vi "ConfigurationPage.vi"(9 "Parameter defaults":string, 10 "Parameters":T1, 11 "Stop":T2) -> ()   [LabVIEW 2020, in "DefaultExtensions.lvlib" / "CGrapherDGML.lvclass"]
uses:
  CGrapherDGML.lvclass
  Private/Parameters.ctl
  obj/Addons/ExtensionInterfaces.lvlibp/IConfigurationPage/Event_Stop.ctl
  obj/Addons/ExtensionInterfaces.lvlibp/IConfigurationPage/IConfigurationPage.lvclass
  obj/Addons/ExtensionInterfaces.lvlibp/IConfigurationPage/Event_StopRef.ctl
  obj/Addons/ExtensionInterfaces.lvlibp/IConfigurationPage/Event_Parameters.ctl
  obj/Addons/ExtensionInterfaces.lvlibp/IConfigurationPage/Event_ParametersRef.ctl
panel:
  in  "Add virtual folders?":bool
  in  "Group by folder":bool
  in  "Expand containers":bool
  in  "Show full paths":bool
  in  "Source folder?":bool
  in  "Target folder?":bool
  in  "Results path":path
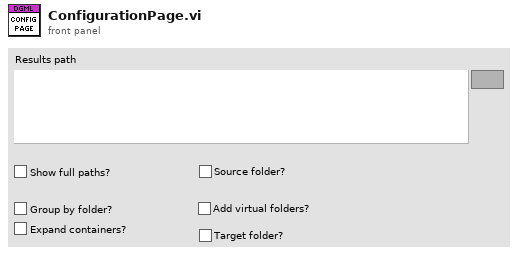
[diagram p1: front panel]
types:
  T1 = typedef "ExtensionInterfaces.lvlibp/IConfigurationPage.lvclass/Event_ParametersRef.ctl" = refnum<user-event>
  T2 = typedef "ExtensionInterfaces.lvlibp/IConfigurationPage.lvclass/Event_StopRef.ctl" = refnum<user-event>
  T3 = typedef "DefaultExtensions.lvlib/CGrapherDGML.lvclass/Parameters.ctl" = cluster{"Path":string, "Expand containers":bool, "Group by folder":bool, "Show full paths":bool, "Source folder?":bool, "Target folder?":bool, "Add virtual folders?":bool}
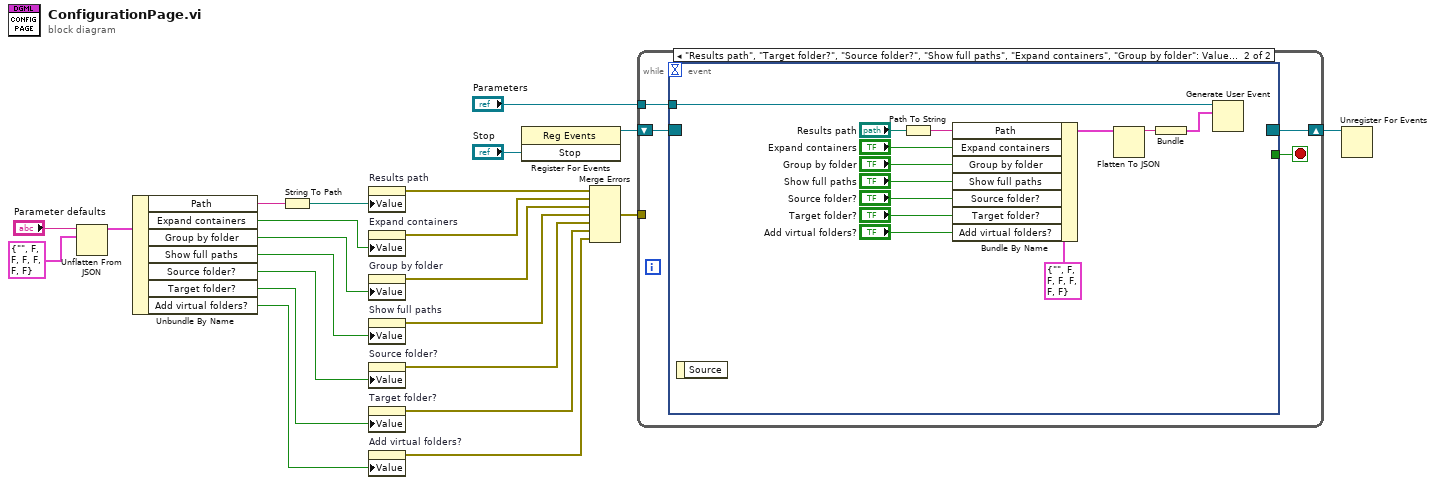
[diagram p0: block diagram]
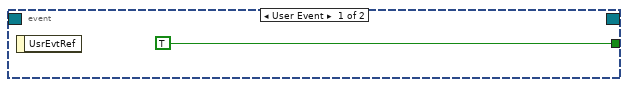
[diagram p2: hidden frame]
diagram:
  n1 = Unflatten From JSON(JSON string="Parameter defaults", type and defaults=T3 {"Path"="", "Expand containers"=FALSE, "Group by folder"=FALSE, "Show full paths"=FALSE, "Source folder?"=FALSE, "Target folder?"=FALSE, "Add virtual folders?"=FALSE} ("Parameters")) -> (value=w17:T3)  [unwired: 5 in, 1 out]
  n2 = Unbundle By Name(w17) -> ("Path"=w16:string, "Expand containers"=w14:bool, "Group by folder"=w13:bool, "Show full paths"=w12:bool, "Source folder?"=w11:bool, "Target folder?"=w10:bool, "Add virtual folders?"=w1:bool)
  n3 = String To Path(string=w16) -> (path=w15:path)
  n4 = property on="Results path" class="Path"("Value"=w15) -> (error out=w9:errorcluster)  [unwired: 2 in, 1 out]
  n5 = property on="Expand containers" class="Bool (strict)"("Value"=w14) -> (error out=w8:errorcluster)  [unwired: 2 in, 1 out]
  n6 = property on="Group by folder" class="Bool (strict)"("Value"=w13) -> (error out=w7:errorcluster)  [unwired: 2 in, 1 out]
  n7 = property on="Show full paths" class="Bool (strict)"("Value"=w12) -> (error out=w6:errorcluster)  [unwired: 2 in, 1 out]
  n8 = property on="Source folder?" class="Bool (strict)"("Value"=w11) -> (error out=w5:errorcluster)  [unwired: 2 in, 1 out]
  n9 = property on="Target folder?" class="Bool (strict)"("Value"=w10) -> (error out=w4:errorcluster)  [unwired: 2 in, 1 out]
  n10 = property on="Add virtual folders?" class="Bool (strict)"("Value"=w1) -> (error out=w2:errorcluster)  [unwired: 2 in, 1 out]
  n11 = register-events("Stop") -> (reference out=w23:refnum<event-registration>)  [unwired: 2 in, 1 out]
  n12 = Merge Errors(w9, w8, w7, w6, w5, w4, w2) -> (w3:errorcluster)
  n13 = while {
    shift-right: [w26] -> w22
    shift-left: w23 -> [w27]
    tunnel: "Parameters" -> [w24]
    tunnel: w3 -> [_]
    stop <- w25 stop-if-true
    n14 = event shown="[1] \"Results path\", \"Target folder?\", \"Source folder?\", \"Show full paths\", \"Expand containers\", \"Group by folder\": Value Change" {
      selector: w27 -> [_ _]
      dyn-events: [_ _] -> w26
      timeout: _ -> [_ _]
      tunnel: [TRUE _] -> w25
      tunnel: w24 -> [_ w37]
      event User Event {
        n15 = event-data() -> ()  [unwired: 1 in, 1 out]
      }
      event "Results path", "Target folder?", "Source folder?", "Show full paths", "Expand containers", "Group by folder": Value Change {
        n16 = event-data() -> ()  [unwired: 1 in, 1 out]
        n17 = Path To String(path="Results path") -> (string=w40:string)
        n18 = Bundle By Name(cluster=T3 {"Path"="", "Expand containers"=FALSE, "Group by folder"=FALSE, "Show full paths"=FALSE, "Source folder?"=FALSE, "Target folder?"=FALSE, "Add virtual folders?"=FALSE} ("Parameters"), "Path"=w40, "Expand containers"="Expand containers", "Group by folder"="Group by folder", "Show full paths"="Show full paths", "Source folder?"="Source folder?", "Target folder?"="Target folder?", "Add virtual folders?"="Add virtual folders?") -> (w41:T3)
        n19 = Flatten To JSON(anything=w41) -> (JSON string=w39:string)  [unwired: 2 in, 1 out]
        n20 = Bundle("JSON string"=w39) -> (w38:cluster{"JSON string":string})  [unwired: 1 in]
        n21 = Generate User Event(user event=w37, event data cluster=w38) -> ()  [unwired: 2 in, 2 out]
      }
    }
  }
  n22 = Unregister For Events(event registration refnum=w22) -> ()  [unwired: 1 in, 1 out]
